vi "NI VeriStand - Close Macro Recorder Reference.vi"(8 "error in (no error)":errorcluster, 11 "MacroRecorder":T1) -> (0 "error out":errorcluster)   [LabVIEW 2020, in "NI_VS MacroRecorderAPI.lvlib"]
doc: "Closes an open reference to the Macro Recorder tool on the VeriStand Gateway. Use this VI to close each <B>MacroRecorder</B> reference that you open with the Open Macro Recorder Reference VI."
uses:
  <vilib>/NI VeriStand/Execution/MacroRecorder/NI_VS MacroRecorderAPI.lvlib
  <vilib>/NI VeriStand/Execution/MacroRecorder/MacroRecorderAPI.ctl
  NationalInstruments.VeriStand.ClientAPI
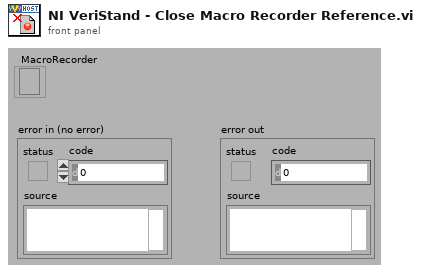
[diagram p1: front panel]
types:
  T1 = typedef "NI_VS MacroRecorderAPI.lvlib/MacroRecorderAPI.ctl" = refnum<k24>
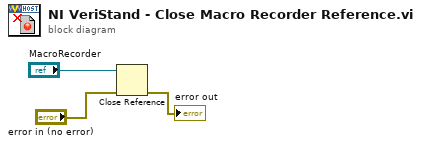
[diagram p0: block diagram]
diagram:
  n1 = Close Reference(reference="MacroRecorder", error in (no error)="error in (no error)") -> (error out=→"error out":errorcluster)
